vi "addTwo.vi"() -> ()   [LabVIEW 2014]
panel:
  out "x+y":dbl
  in  "Numeric":dbl
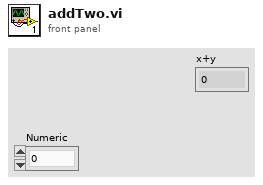
[diagram p1: front panel]
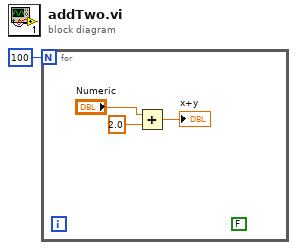
[diagram p0: block diagram]
diagram:
  n1 = for {
    N: 100 -> [_]
    (unwired) FALSE
    n2 = Add(x="Numeric", y=2.0) -> (x+y=→"x+y":dbl)
  }
